vi "unique_name.vi"(11 "Array":dbl[](array[numeric])) -> (1 "Order Index":i16[](array[numeric]), 3 "Unduplicated Array":dbl[](array[numeric]))   [LabVIEW 2015]
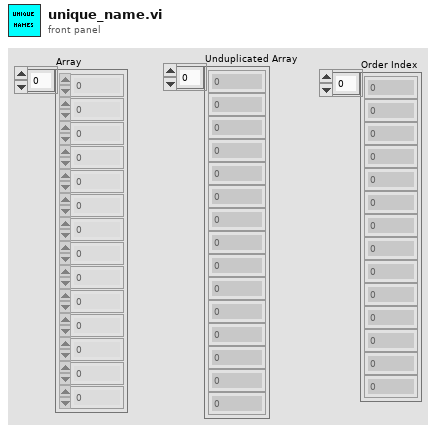
[diagram p1: front panel]
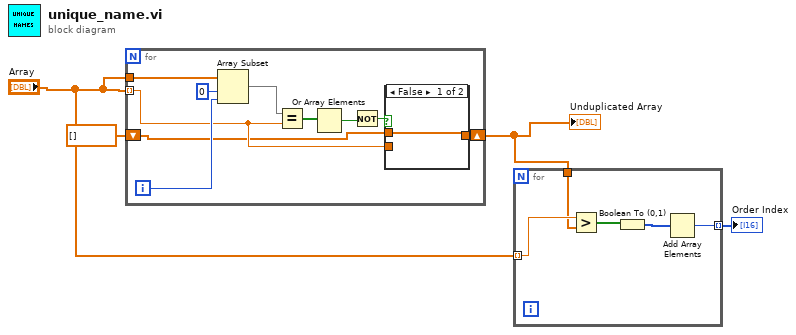
[diagram p0: block diagram]
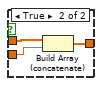
[diagram p2: hidden frame]
diagram:
  n1 = for {
    tunnel: "Array" -> [w7] mode=indexing
    tunnel: "Array" -> [w14]
    shift-right: [w6] -> w2
    shift-left: dbl[] [] -> [w5]
    i -> [w12]
    n2 = Array Subset(array=w14, index=0, length=w12) -> (w11:dbl[])
    n3 = Equal?(x=w11, y=w7) -> (x = y?=w10:bool[])
    n4 = Or Array Elements(Boolean array=w10) -> (logical OR=w9:bool)
    n5 = Not(x=w9) -> (.not. x?=w8:bool)
    n6 = case shown="False" w8 {
      tunnel: w7 -> [_ w18]
      tunnel: [w15 w17] -> w6
      tunnel: w5 -> [w15 w16]
      frame False {
      }
      frame True {
        n7 = Build Array (concatenate)(w16, w18) -> (w17:dbl[])
      }
    }
  }
  "Unduplicated Array" <- w2
  n8 = for {
    tunnel: "Array" -> [w23] mode=indexing
    tunnel: w2 -> [w22]
    tunnel: [w19] -> w1 mode=indexing
    n9 = Greater?(x=w23, y=w22) -> (0:w21:bool[])
    n10 = Boolean To (0,1)(Boolean=w21) -> (0, 1=w20:i16[])
    n11 = Add Array Elements(numeric array=w20) -> (sum=w19:i16)
  }
  "Order Index" <- w1
